vi "Read Hardware Position.vi"(8 "error in (no error)":errorcluster, 10 "SLSC Session in":refnum<class "SLSC Interface.lvclass">, 11 "Relay in":refnum<class "Relay.lvclass">) -> (0 "error out":errorcluster, 2 "RelayPosition":T1=10 caption="position" items=["Open"=10, "Closed"=11], 3 "Relay out":refnum<class "Relay.lvclass">)   [LabVIEW 2015, in "SLSC Switch.lvlib" / "Relay.lvclass"]
uses:
  Relay.lvclass
  slscsl/RelayPosition.ctl
  slscsl/slscsl.lvclass
  <vilib>/National Instruments/SLSC Local or Remote Interface/SLSC Interface Class/SLSC Interface.lvclass
  <vilib>/National Instruments/SLSC Local or Remote Interface/SLSC Interface Class/Get Generic Property/Get Generic Property (Bool).vi
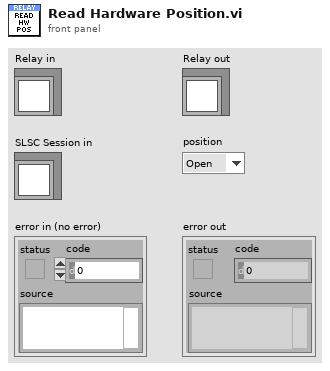
[diagram p1: front panel]
types:
  T1 = typedef "SLSC Switch.lvlib/slscsl.lvclass/RelayPosition.ctl" = i32
  T2 = typedef "SLSC Switch.lvlib/Relay.lvclass/Property.ctl" = cluster{"resource name":string, "property":refnum<k21>}
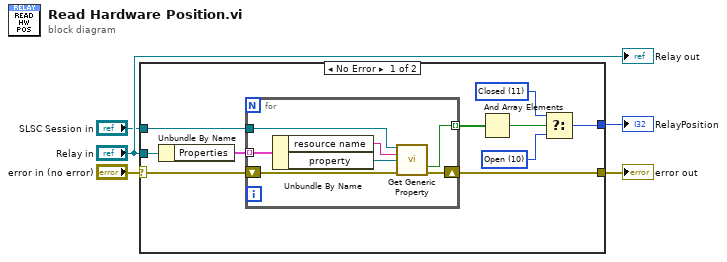
[diagram p0: block diagram]
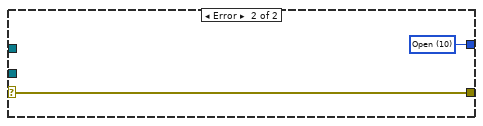
[diagram p2: hidden frame]
diagram:
  n1 = case shown="No Error" "error in (no error)" {
    selector: "error in (no error)" -> [w14 w24]
    tunnel: [w13 w24] -> w4
    tunnel: "Relay in" -> [w15 _]
    tunnel: [w10 w23] -> w2
    tunnel: "SLSC Session in" -> [w6 _]
    frame No Error {
      w11 = T1 10 items=["Open"=10, "Closed"=11] ("f")
      w12 = T1 11 items=["Open"=10, "Closed"=11] ("RelayPosition")
      n2 = Unbundle By Name(w15) -> ("Properties"=w9:T2[])
      n3 = for {
        shift-right: [w20] -> w13
        shift-left: w14 -> [w21]
        tunnel: w9 -> [w22] mode=indexing
        tunnel: [w19] -> w7 mode=indexing
        tunnel: w6 -> [w16]
        n4 = Unbundle By Name(w22) -> ("resource name"=w18:string, "property"=w17:refnum<k21>)
        n5 = call-poly <vilib>:"Get Generic Property.vi"("SLSC Interface in"=w16, "resources"=w18, "property"=w17, "error in (no error)"=w21) -> ("property value"=w19:bool, "error out"=w20:errorcluster)  [unwired: 9 in, 1 out]
      }
      n6 = And Array Elements(Boolean array=w7) -> (logical AND=w8:bool)
      n7 = Select(t=w12, s=w8, f=w11) -> (s? t:f=w10:T1)
    }
    frame Error {
      w23 = T1 10 items=["Open"=10, "Closed"=11] ("f")
    }
  }
  "error out" <- w4
  "RelayPosition" <- w2
  "Relay out" <- "Relay in"
